vi "FRCts20_WebMethods_Division_POST.vi"(7 "httpRequestID":u32, 11 "competition":string) -> ()   [LabVIEW 2014, in "FRCts20_WebMethods.lvlib"]
doc: "<B>POST</B> a new division resource\n\n<B>Required XML Data : </B>\n<Division>\n <Location><B>string</B></Location>\n</Division>\n\nhttp://<server address>:<port>/FRCts/competition/<B>competition</B>/division/\n\n{requires authentication}"
uses:
  FRCts20_WebMethods.lvlib
  <vilib>/wsapi/NI_WebServices.lvlib
  Backend/source/VI Source/FRCts20_Backend_API/FRCts20_Backend_API.lvlib
  Backend/source/VI Source/FRCts20_Backend_API/FRCts20_Backend_API_SW.ctl
  Backend/source/VI Source/FRCts20_Backend_API/FRCts20_Backend_API_Division.ctl
  Backend/source/VI Source/FRCts20_Backend_API/FRCts20_Backend_API_Command_Division.ctl
  FRCts20_WebMethods_ReadData_Division.vi
  Backend/source/VI Source/FRCts20_Backend_API/FRCts20_Backend_API_Status.ctl
  Backend/source/VI Source/FRCts20_Backend_API/FRCts20_Backend_API_Application.vi
  FRCts20_WebMethods_Redirect_Request.vi
panel:
  in  "query":string
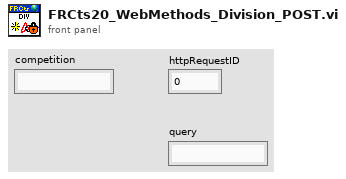
[diagram p1: front panel]
types:
  T1 = typedef "FRCts20_Backend_API.lvlib/FRCts20_Backend_API_Division.ctl" = cluster{"Location":string, "Team":u32[], "APIReturn":string, "RootCmd":enum16{"Issues", "Software", "All"}, "SWType":T2, "Status":T3, "Competition":string}
  T2 = typedef "FRCts20_Backend_API.lvlib/FRCts20_Backend_API_SW.ctl" = string
  T3 = typedef "FRCts20_Backend_API.lvlib/FRCts20_Backend_API_Status.ctl" = enum16{"Open", "In Work", "Closed"}
  T4 = typedef "FRCts20_Backend_API.lvlib/FRCts20_Backend_API_Command_Division.ctl" = string
  T5 = typedef "FRCts20_Backend_API.lvlib/FRCts20_Backend_API_Application.ctl" = cluster{"Revision":string, "APIReturn":string}
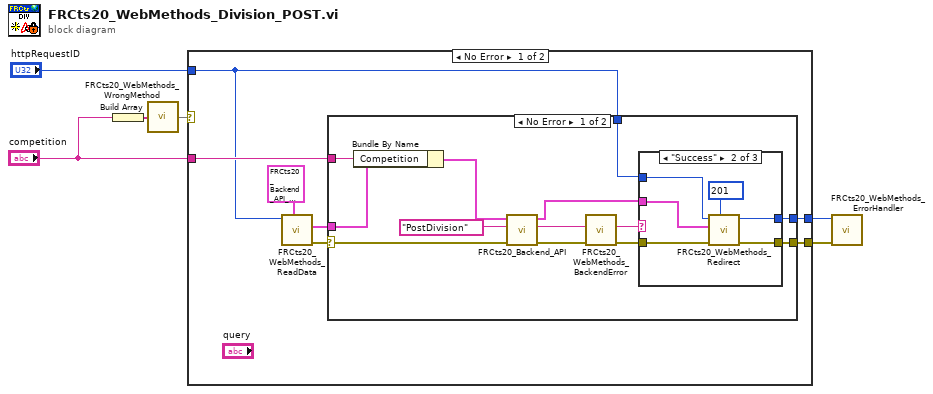
[diagram p0: block diagram]
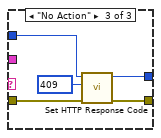
[diagram p3: hidden frame]
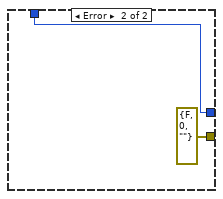
[diagram p4: hidden frame]
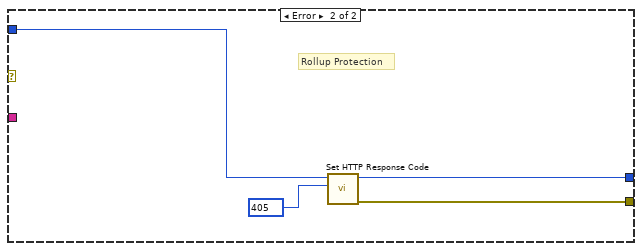
[diagram p5: hidden frame]
diagram:
  n1 = Build Array("competition") -> (w5:string[])
  n2 = call "FRCts20_WebMethods_WrongMethod.vi"(4:w5) -> (1:w6)  [unwired: 3 in, 1 out]
  n3 = case shown="No Error" w6 {
    tunnel: "httpRequestID" -> [w8 w45]
    tunnel: [w11 w43] -> w2
    tunnel: [w12 w42] -> w3
    tunnel: "competition" -> [w13 _]
    frame No Error {
      n4 = call-poly "FRCts20_WebMethods_ReadData.vi"("Cluster Type"=T1 {"Location"="", "Team"=[], "APIReturn"="", "RootCmd"=enum."Issues", "SWType"="", "Status"=enum."Open", "Competition"=""} ("Division"), "httpRequestID"=w8) -> ("error out"=w7:errorcluster, "Cluster out"=w9:T1)  [unwired: 7 in, 1 out]
      n5 = case shown="No Error" w7 {
        selector: w7 -> [w14 _]
        tunnel: w13 -> [w26 _]
        tunnel: [w18 errorcluster {"status"=FALSE, "code"=0, "source"=""} ("error out")] -> w12
        tunnel: [w17 w40] -> w11
        tunnel: w9 -> [w16 _]
        tunnel: w8 -> [w15 w40]
        frame No Error {
          n6 = Bundle By Name(cluster=w16, "Competition"=w26) -> (w25:T1)
          n7 = call-poly "FRCts20_Backend_API.vi"("error in (no error)"=w14, "Command"=T4 "PostDivision", 11:w25) -> ("error out"=w23:errorcluster, "Status"=w22:string, "Application"=w19:T5)  [unwired: 6 in]
          n8 = call "FRCts20_WebMethods_BackendError.vi"("error in (no error)"=w23, "Status"=w22) -> ("error out"=w21:errorcluster, "Status out"=w20:string)  [unwired: 8 in]
          n9 = case shown="\"Success\"" w20 {
            tunnel: w21 -> [w27 w34 w36]
            tunnel: w19 -> [_ w30 _]
            tunnel: w15 -> [w28 w31 w37]
            tunnel: [w27 w32 w39] -> w18
            tunnel: [w28 w33 w38] -> w17
            frame "Backend Error", Default {
            }
            frame "Success" {
              w29 = 201 items=["100"=100, "101"=101, "200"=200, "201"=201, "202"=202, "203"=203, "204"=204, "205"=205, "206"=206, "300"=300, "301"=301, "302"=302, "303"=303, "304"=304, "305"=305, "306"=306, "307"=307, "400"=400, "401"=401, "402"=402, "403"=403, "404"=404, "405"=405, "406"=406, "407"=407, "408"=408, "409"=409, "410"=410, "411"=411, "412"=412, "413"=413, "414"=414, "415"=415, "416"=416, "417"=417, "500"=500, "501"=501, "502"=502, "503"=503, "504"=504, "505"=505] ("response code (200)")
              n10 = call-poly "FRCts20_WebMethods_Redirect.vi"("response code (200)"=w29, "error in (no error)"=w34, "Request"=w30, "httpRequestID"=w31) -> ("error out"=w32:errorcluster, "httpRequestID out"=w33:u32)  [unwired: 6 in]
            }
            frame "No Action" {
              w35 = 409 items=["100"=100, "101"=101, "200"=200, "201"=201, "202"=202, "203"=203, "204"=204, "205"=205, "206"=206, "300"=300, "301"=301, "302"=302, "303"=303, "304"=304, "305"=305, "306"=306, "307"=307, "400"=400, "401"=401, "402"=402, "403"=403, "404"=404, "405"=405, "406"=406, "407"=407, "408"=408, "409"=409, "410"=410, "411"=411, "412"=412, "413"=413, "414"=414, "415"=415, "416"=416, "417"=417, "500"=500, "501"=501, "502"=502, "503"=503, "504"=504, "505"=505] ("response code (200)")
              n11 = call <vilib>:"Set HTTP Response Code.vi"("error in (no error)"=w36, "response code (200)"=w35, "httpRequestID"=w37) -> ("error out"=w39:errorcluster, "httpRequestID out"=w38:u32)  [unwired: 7 in]
            }
          }
        }
        frame Error {
        }
      }
    }
    frame Error {
      w44 = 405 items=["100"=100, "101"=101, "200"=200, "201"=201, "202"=202, "203"=203, "204"=204, "205"=205, "206"=206, "300"=300, "301"=301, "302"=302, "303"=303, "304"=304, "305"=305, "306"=306, "307"=307, "400"=400, "401"=401, "402"=402, "403"=403, "404"=404, "405"=405, "406"=406, "407"=407, "408"=408, "409"=409, "410"=410, "411"=411, "412"=412, "413"=413, "414"=414, "415"=415, "416"=416, "417"=417, "500"=500, "501"=501, "502"=502, "503"=503, "504"=504, "505"=505] ("response code (200)")
      # "Rollup Protection"
      n12 = call <vilib>:"Set HTTP Response Code.vi"("response code (200)"=w44, "httpRequestID"=w45) -> ("error out"=w42:errorcluster, "httpRequestID out"=w43:u32)  [unwired: 8 in]
    }
  }
  n13 = call "FRCts20_WebMethods_ErrorHandler.vi"("error in"=w3, "httpRequestID"=w2) -> ()  [unwired: 9 in, 1 out]
